vi "Test Process Register For Broadcast Throws Error if Process Uninitialized.vi"(8 "error in (no error)":errorcluster, 11 "Process Test in":refnum<class "Process Test.lvclass">) -> (0 "error out":errorcluster, 3 "Process Test out":refnum<class "Process Test.lvclass">)   [LabVIEW 2020, in "Process Test.lvclass"]
uses:
  Process Test.lvclass
  Framework/Process/Process.lvclass
  <vilib>/Asteme/LUnit/Test Case.lvclass
  C:/Users/anton/Documents/GitHub/Triarc-Framework/source/Framework Test/Base Class Test/Base Test.lvclass
  C:/Program Files (x86)/National Instruments/LabVIEW 2020/vi.lib/Asteme/LUnit/Test Case.lvclass
  C:/Users/anton/Documents/GitHub/Triarc-Framework/source/Framework Test/Process Test/Process Test.lvclass
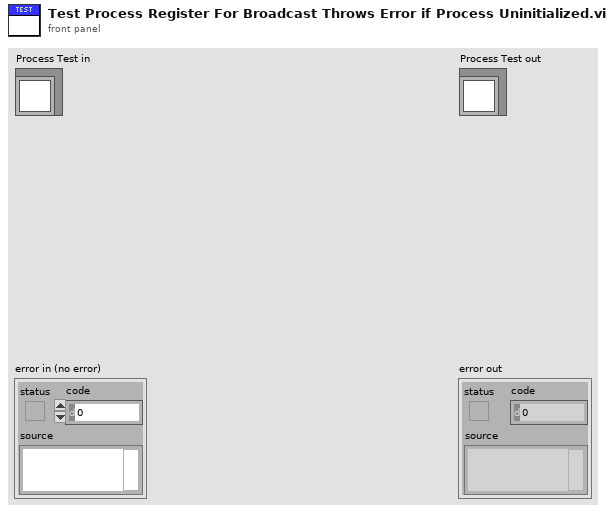
[diagram p1: front panel]
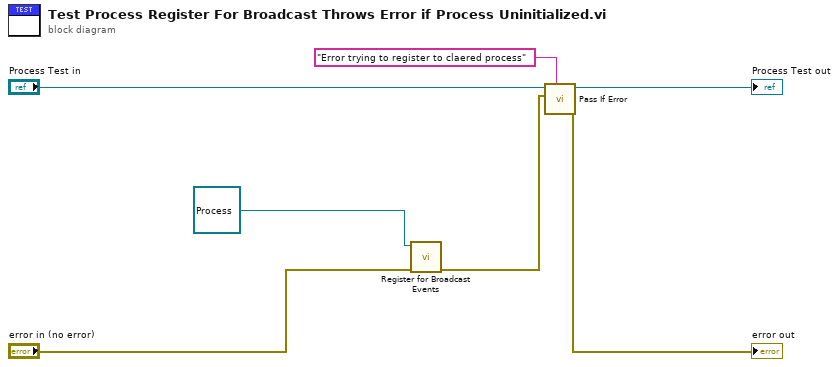
[diagram p0: block diagram]
diagram:
  n1 = call "Register for Broadcast Events.vi"("error in (no error)"="error in (no error)", "Process In"=refnum<class "Process.lvclass"> refnum ("Process.lvclass")) -> ("error out"=w2:errorcluster)  [unwired: 7 in, 2 out]
  n2 = call <vilib>:"Pass If Error.vi"("Description"="Error trying to register to claered process", "Assert error"=w2, "Test Case In"="Process Test in") -> ("error out"=→"error out":errorcluster, "Test Case Out"=→"Process Test out":refnum<class "Process Test.lvclass">)  [unwired: 7 in]
